vi "Zhiyuan ZDS Serial Read Scope Bitmap.vi"() -> ()   [LabVIEW 2015]
doc: "This example shows how to read scope bitmap."
uses:
  ZhiYuan ZDS Series for TCP.lvlib
panel:
  out "scope bmp":picture
  in  "VISA resource name":refnum<visa-resource-name>
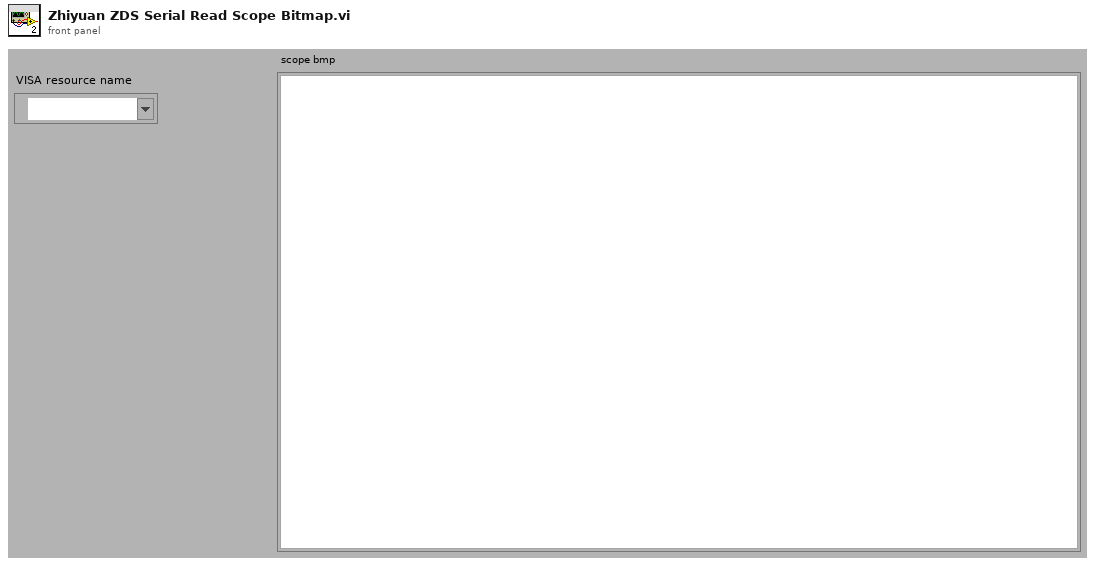
[diagram p1: front panel]
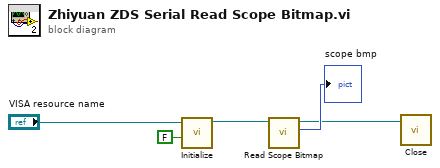
[diagram p0: block diagram]
diagram:
  n1 = call "Initialize.vi"("Reset (True)"=FALSE, "VISA resource name"="VISA resource name") -> ("VISA resource name out"=w4:refnum<visa-resource-name>)  [unwired: 8 in, 1 out]
  n2 = call "Read Scope Bitmap.vi"("VISA resource name"=w4) -> ("scope"=→"scope bmp":picture, "VISA resource name out"=w2:refnum<visa-resource-name>)  [unwired: 8 in, 1 out]
  n3 = call "Close.vi"("VISA resource name"=w2) -> ()  [unwired: 10 in, 1 out]
